vi "Demo.vi"() -> ()   [LabVIEW 2019, in "BlueTOMLSerializer.lvlib"]
uses:
  BlueTOMLSerializer.lvlib
  <userlib>/Blue Origin/BlueSerialization/BlueSerializer/BlueSerializer.lvclass
panel:
  out "equal?":bool
  out "error out":errorcluster
  out "TOML 2":string
  out "TOML 1":string
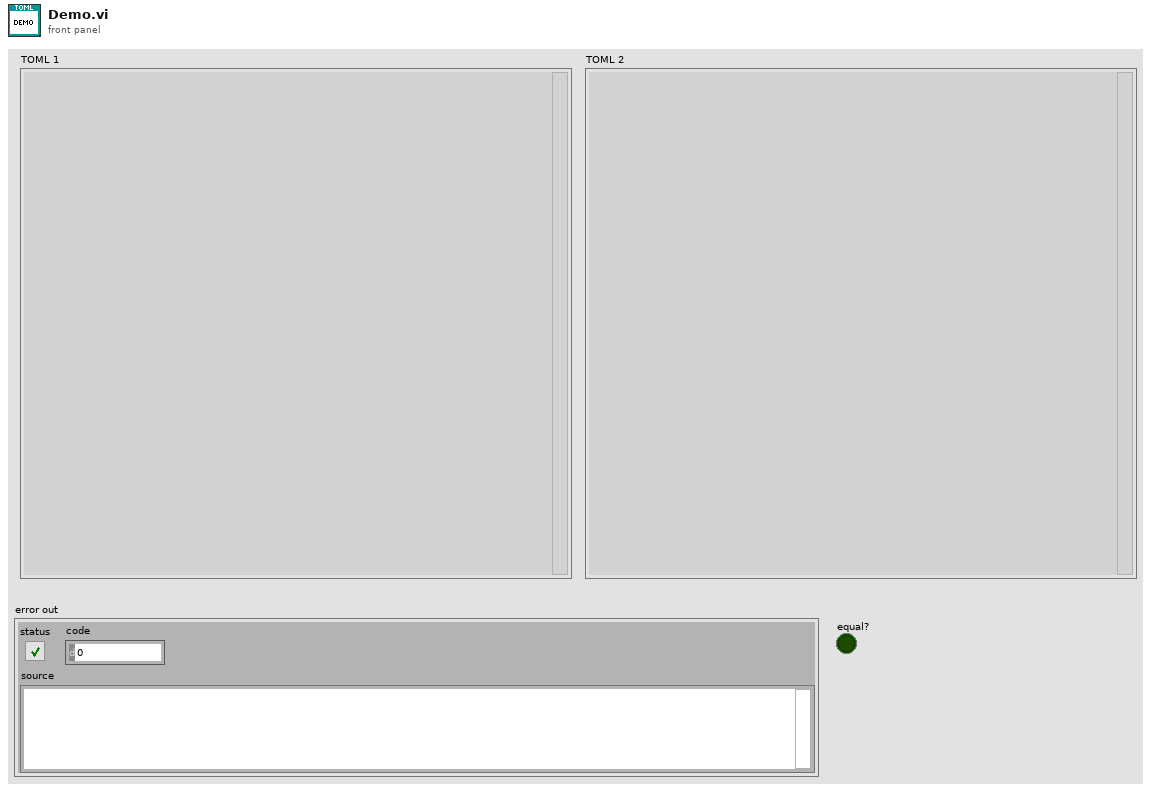
[diagram p1: front panel]
types:
  T1 = cluster{"Name":string, "CarNumber":i32, "LapRecords":cluster{"Track":string, "FastestLap":dbl, "Car":cluster{"Sponsor":string, "S/N":i32}}[], "HallOfFame":cluster{"HallOfFame?":bool, "YearInducted":timestamp}}
  T2 = typedef "BlueTOMLSerializer.lvlib/TOML Value.ctl" = cluster{"\\type":enum16{"Table", "Array", "String", "Integer", "Float", "Boolean", "Offset Date-Time", "Local Date-Time", "Local Date", "Local Time"}, "ÿýÿýÿýÿýÿýÿþÿýÿýÿý%LV-TOML.lvlib:TOML Key-Value Pair.ctlÿýÿýÿýÿýÿýÿþÿýÿýÿýLV-TOML.lvlib:TOML Value.ctl$":variant}
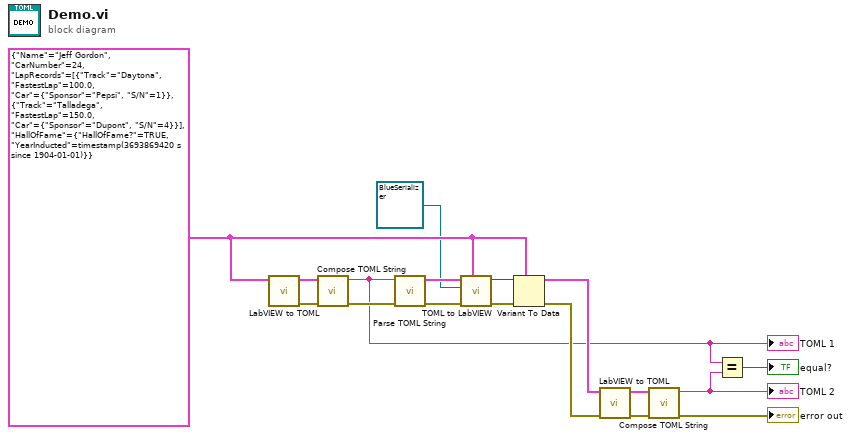
[diagram p0: block diagram]
diagram:
  w10 = T1 {"Name"="Jeff Gordon", "CarNumber"=24, "LapRecords"=[{"Track"="Daytona", "FastestLap"=100.0, "Car"={"Sponsor"="Pepsi", "S/N"=1}}, {"Track"="Talladega", "FastestLap"=150.0, "Car"={"Sponsor"="Dupont", "S/N"=4}}], "HallOfFame"={"HallOfFame?"=TRUE, "YearInducted"=timestamp(3693869420.6870832 s since 1904-01-01)}}
  n1 = call "LabVIEW to TOML.vi"("LV Value"=w10) -> ("error out"=w15:errorcluster, "TOML Value"=w16:T2)  [unwired: 9 in]
  n2 = call "Compose TOML String.vi"("error in (no error)"=w15, "Value"=w16) -> ("error out"=w14:errorcluster, "String"=w3:string)  [unwired: 8 in]
  "TOML 1" <- w3
  n3 = call "Parse TOML String.vi"("error in (no error)"=w14, "String"=w3) -> ("error out"=w13:errorcluster, "Value"=w17:T2)  [unwired: 8 in]
  n4 = call "TOML to LabVIEW.vi"("Default Value"=w10, "error in (no error)"=w13, "BlueSerializer in"=refnum<class "BlueSerializer.lvclass"> refnum, "TOML Value"=w17) -> ("error out"=w12:errorcluster, "LV Value"=w11:variant)  [unwired: 6 in]
  n5 = Variant To Data(error in=w12, type=w10, Variant=w11) -> (data=w5:T1, error out=w7:errorcluster)
  n6 = call "LabVIEW to TOML.vi"("error in (no error)"=w7, "LV Value"=w5) -> ("error out"=w9:errorcluster, "TOML Value"=w8:T2)  [unwired: 8 in]
  n7 = call "Compose TOML String.vi"("error in (no error)"=w9, "Value"=w8) -> ("error out"=→"error out":errorcluster, "String"=w4:string)  [unwired: 8 in]
  "TOML 2" <- w4
  n8 = Equal?(x=w3, y=w4) -> (x = y?=→"equal?":bool)
